vi "Enable Controls.vi"(8 "error in (no error)":errorcluster, 10 "Number of Enabled Controls":i32, 11 "Controls":refnum<vi>[](array[refnum])) -> (0 "error out":errorcluster, 3 "dup Controls":refnum<vi>[](array[refnum]))   [LabVIEW 2024]
doc: "Enables a given number of the controls on the front panel."
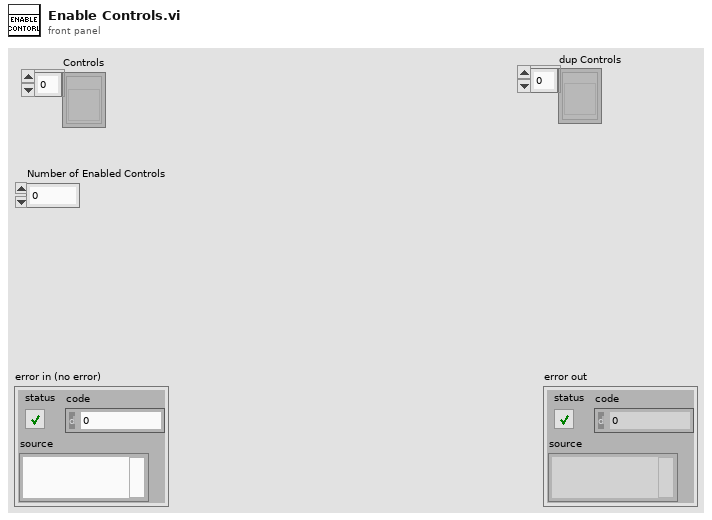
[diagram p1: front panel]
types:
  T1 = enum8{"Enabled", "Disabled", "Disabled and Grayed Out"}
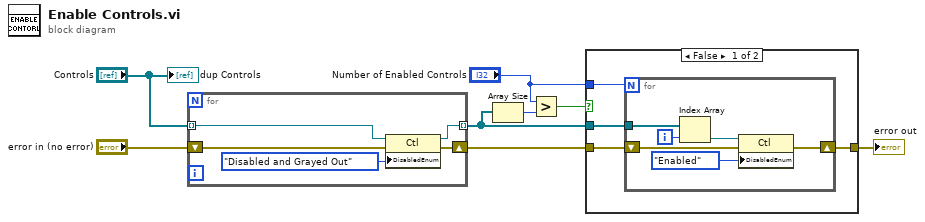
[diagram p0: block diagram]
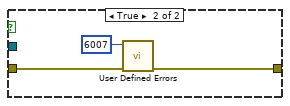
[diagram p2: hidden frame]
diagram:
  n1 = for {
    tunnel: "Controls" -> [w13] mode=indexing
    tunnel: [w12] -> w4 mode=indexing
    shift-right: [w11] -> w1
    shift-left: "error in (no error)" -> [w10]
    n2 = property class="Ctl"(reference=w13, error in=w10, "DisabledEnum"=T1."Disabled and Grayed Out" ("Disabled")) -> (reference out=w12:refnum<vi>, error out=w11:errorcluster)
  }
  n3 = Array Size(array=w4) -> (size(s)=w3:i32)
  n4 = Greater?(x="Number of Enabled Controls", y=w3) -> (0:w2:bool)
  n5 = case shown="False" w2 {
    tunnel: w4 -> [w17 _]
    tunnel: "Number of Enabled Controls" -> [w16 _]
    tunnel: w1 -> [w15 w25]
    tunnel: [w14 w24] -> w7
    frame False {
      n6 = for {
        N: w16 -> [_]
        tunnel: w17 -> [w23]
        shift-right: [w19] -> w14
        shift-left: w15 -> [w18]
        i -> [w22]
        n7 = Index Array(array=w23, index=w22) -> (element=w21:refnum<vi>)
        n8 = property class="Ctl"(reference=w21, error in=w18, "DisabledEnum"=T1."Enabled" ("Disabled")) -> (error out=w19:errorcluster)  [unwired: 1 out]
      }
    }
    frame True {
      n9 = call "User Defined Errors.vi"("error in (no error)"=w25, "Error Code (0)"=6007 ("error code (0)")) -> ("error out"=w24:errorcluster)  [unwired: 9 in]
    }
  }
  "error out" <- w7
  "dup Controls" <- "Controls"
